vi "Solve1.vi"(8 "Error In":errorcluster, 11 "object in":refnum<class "2021_16.lvclass">) -> (0 "Error Out":errorcluster, 2 "Result":u64, 3 "object out":refnum<class "2021_16.lvclass">)   [LabVIEW 2023, in "2021_16.lvclass"]
uses:
  2021_16.lvclass
  2021_16.lvclass/2021_16.ctl
  <userlib>/_OpenG.lib/string/string.llb/openg_string.lvlib
  16_Helper_class/16_Helper.lvclass
panel:
  out "literal value":u64
  # "556 too high"
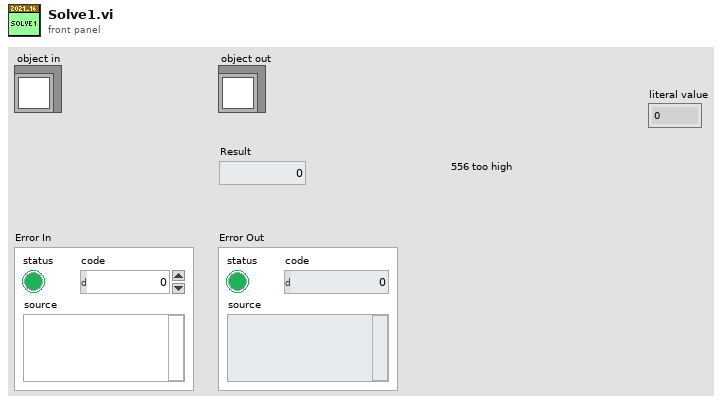
[diagram p1: front panel]
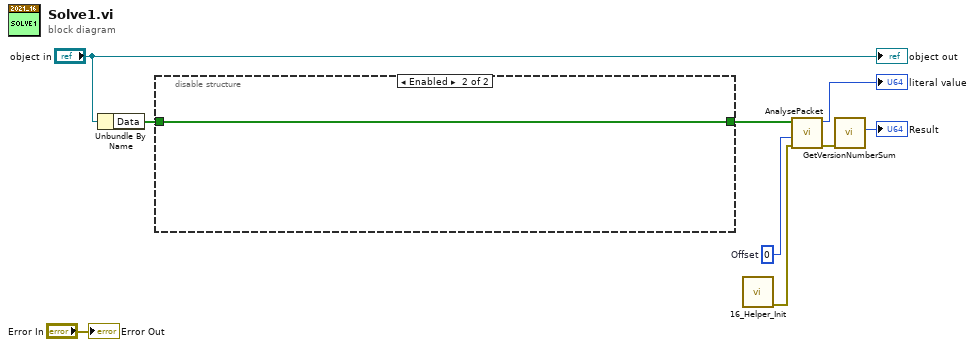
[diagram p0: block diagram]
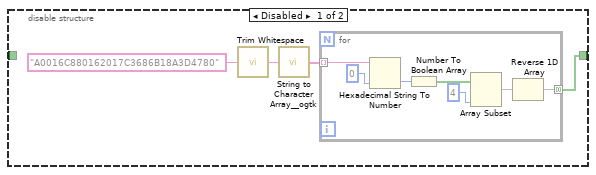
[diagram p2: hidden frame]
diagram:
  w6 = 0  # Offset
  n1 = Unbundle By Name("object in") -> ("Data"=w1:bool[])
  n2 = disable-structure shown="Enabled" {
    disable-tunnel: [w10 w21] -> w7
    disable-tunnel: w1 -> [_ w21]
    frame Disabled {
      n3 = call <vilib>:"Trim Whitespace.vi"("string"="A0016C880162017C3686B18A3D4780") -> ("trimmed string"=w13:string)  [unwired: 1 in]
      n4 = call <userlib>:"String to Character Array__ogtk.vi"("Input String"=w13) -> ("Character Array"=w12:string[])
      n5 = for {
        tunnel: w12 -> [w20] mode=indexing
        tunnel: [w14] -> w10 mode=concatenating
        n6 = Hexadecimal String To Number(string=w20, default (0uL)=u8 0 ("default (0 U32)")) -> (number=w18:u8)  [unwired: 1 in, 1 out]
        n7 = Number To Boolean Array(number=w18) -> (Boolean array=w17:bool[])
        n8 = Array Subset(array=w17, length=4) -> (w15:bool[])  [unwired: 1 in]
        n9 = Reverse 1D Array(array=w15) -> (reversed array=w14:bool[])
      }
    }
    frame Enabled {
    }
  }
  n10 = call "16_Helper_Init.vi"() -> ("Error Out"=w4:errorcluster)  [unwired: 10 in, 1 out]
  n11 = call "AnalysePacket.vi"("error in"=w4, "Offset"=w6, "Data"=w7) -> ("error out"=w3:errorcluster, "Result"=→"literal value":u64)  [unwired: 6 in, 1 out]
  n12 = call "GetVersionNumberSum.vi"("Error In"=w3) -> ("VersionNumberSum"=→"Result":u64)  [unwired: 9 in, 1 out]
  "Error Out" <- "Error In"
  "object out" <- "object in"
